vi "get channel names from typedef.vi"(8 "error in":errorcluster, 10 "channel classification":T1, 11 "fixed channel configuration":refnum<class "fixed channel configuration.lvclass">) -> (0 "error out":errorcluster, 3 "Channel Names":string[](array[string]))   [LabVIEW 2013, in "fixed channel configuration.lvclass"]
uses:
  fixed channel configuration.lvclass
  <vilib>/NI/Tag Bus Module Framework/channel/channel classification.ctl
  <vilib>/Utility/VariantDataType/VariantType.lvlib
  <vilib>/NI/Tag Bus Module Framework/channel/TBM channel.lvclass
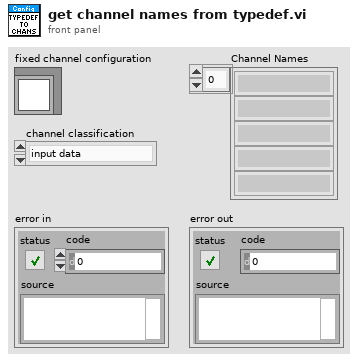
[diagram p1: front panel]
types:
  T1 = typedef "TBM channel.lvclass/channel classification.ctl" = enum16{"input data", "output data", "processing parameter", "processing result"}
  T2 = typedef "fixed channel configuration.lvclass/index type definitions.ctl" = cluster{"input indices":variant, "parameter indices":variant, "result indices":variant, "output indices":variant}
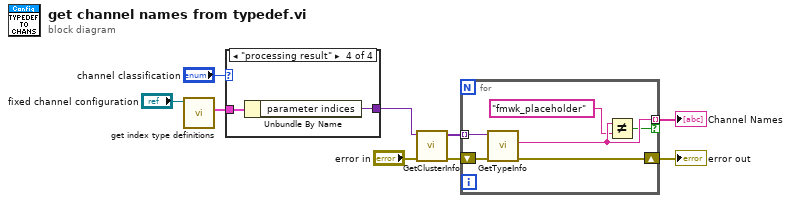
[diagram p0: block diagram]
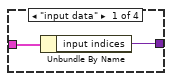
[diagram p2: hidden frame]
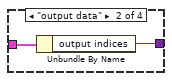
[diagram p3: hidden frame]
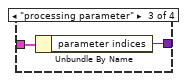
[diagram p4: hidden frame]
diagram:
  n1 = call-dynamic "get index type definitions.vi"("fixed channel configuration in"="fixed channel configuration") -> ("index type defs"=w1:T2)  [unwired: 9 in, 1 out]
  n2 = case shown="\"processing result\"" "channel classification" {
    tunnel: [w10 w12 w14 w16] -> w5
    tunnel: w1 -> [w11 w13 w15 w17]
    frame "input data" {
      n3 = Unbundle By Name(w11) -> ("input indices"=w10:variant)
    }
    frame "output data" {
      n4 = Unbundle By Name(w13) -> ("output indices"=w12:variant)
    }
    frame "processing parameter" {
      n5 = Unbundle By Name(w15) -> ("parameter indices"=w14:variant)
    }
    frame "processing result" {
      n6 = Unbundle By Name(w17) -> ("parameter indices"=w16:variant)
    }
  }
  n7 = call <vilib>:"GetClusterInfo.vi"("error in (no error)"="error in", "Variant"=w5) -> ("error out"=w7:errorcluster, "Cluster Elements"=w8:variant[])  [unwired: 8 in]
  n8 = for {
    tunnel: w8 -> [w23] mode=indexing
    tunnel: [w20] -> w3 mode=indexing if=w19
    shift-right: [w22] -> w4
    shift-left: w7 -> [w21]
    n9 = call <vilib>:"GetTypeInfo.vi"("error in (no error)"=w21, "Variant"=w23) -> ("error out"=w22:errorcluster, "Name"=w20:string)  [unwired: 5 in, 3 out]
    n10 = Not Equal?(x=w20, y="fmwk_placeholder") -> (x != y?=w19:bool)
  }
  "Channel Names" <- w3
  "error out" <- w4
